vi "Get DUT Setup Parameters.vi"(8 "error in (no error)":errorcluster, 11 "QPA Measurement in":refnum<class "QPA Measurement.lvclass">) -> (0 "error out":errorcluster, 3 "QPA Measurement out":refnum<class "QPA Measurement.lvclass">)   [LabVIEW 2016, in "QPA Measurement.lvlib" / "QPA Measurement.lvclass"]
uses:
  QPA Measurement.lvclass
  C:/Projects/STS/Common/Sequence Automation/Plugins/Measurement Interface.lvlibp/Measurement Interface.lvclass
  QPA Measurement.lvclass/QPA Measurement.ctl
  Controls/Parameter.ctl
  Plugins/Measurement Interface.lvlibp/Private Methods/Active Sequence File/Read Active Sequence File.vi
  Plugins/TestStand API Tools (TSAT).lvlibp/Sequence File Actions/TSAT Sequence File Actions.lvlib
  Plugins/TestStand API Tools (TSAT).lvlibp/Sequence Actions/TSAT Sequence Actions.lvlib
  Plugins/TestStand API Tools (TSAT).lvlibp/TSAT Utilities/TSAT Utilities.lvlib
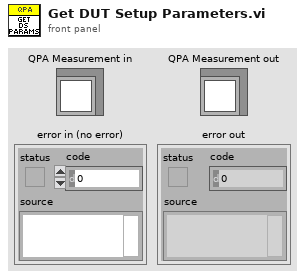
[diagram p1: front panel]
types:
  T1 = enum16{"Container", "String", "Boolean", "Number", "NamedType", "Reference", "Array", "Aperture Time"}
  T2 = typedef "QPA Measurement.lvlib/QPA Measurement.lvclass/Parameter.ctl" = cluster{"Name":string, "PropertyObject Type":enum16{"Container", "String", "Boolean", "Number", "NamedType", "Reference", "Array", "Aperture Time"}}
  T3 = enum16{"Container", "String", "Boolean", "Number", "NamedType", "Reference", "Array"}
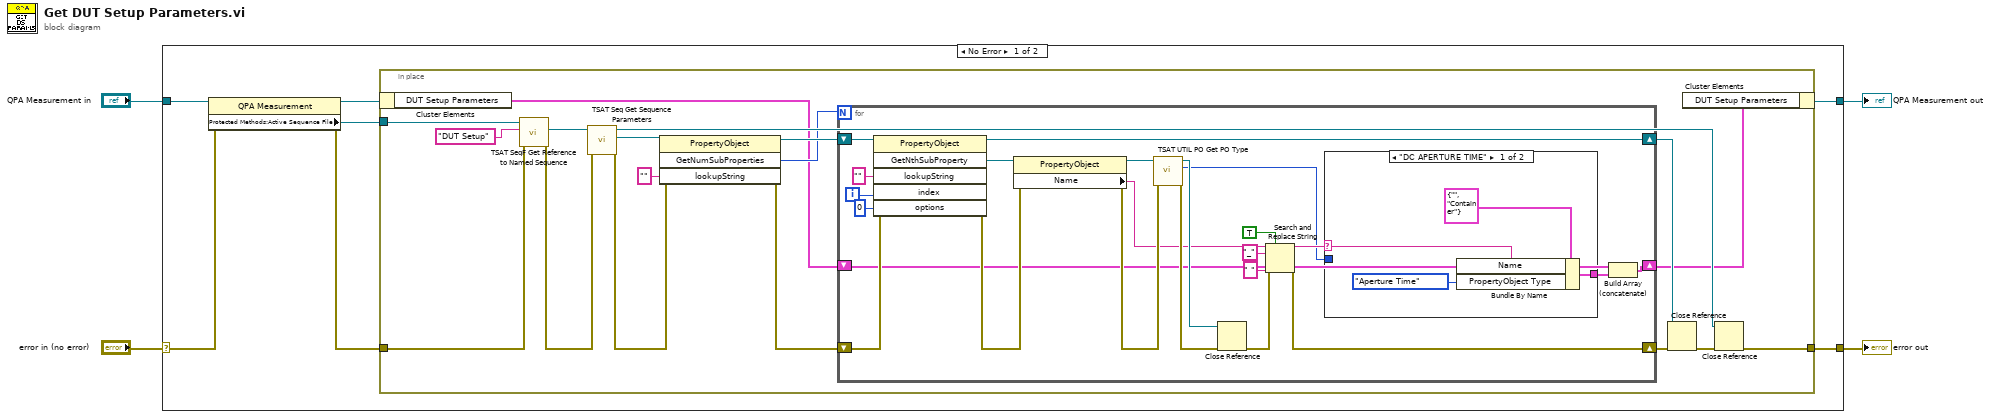
[diagram p0: block diagram]
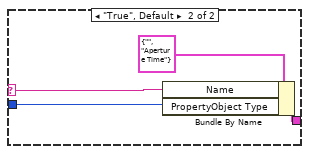
[diagram p2: hidden frame]
diagram:
  n1 = case shown="No Error" "error in (no error)" {
    selector: "error in (no error)" -> [w11 w62]
    tunnel: [w5 w62] -> w3
    tunnel: [w10 w61] -> w1
    tunnel: "QPA Measurement in" -> [w8 w61]
    frame No Error {
      n2 = property class="QPA Measurement"(reference=w8, error in=w11) -> (reference out=w7:refnum<class "QPA Measurement.lvclass">, error out=w9:errorcluster, "Protected Methods:Active Sequence File"=w6:refnum<k7>)
      n3 = in-place {
        in-place-border: w9 -> [w28]
        in-place-border: w6 -> [w29]
        in-place-border: [w16] -> w5
        n4 = in-place-cluster #1(w7) -> ("DUT Setup Parameters"=w13:T2[])
        n5 = call "TSAT SeqF Get Reference to Named Sequence.vi"("Error In"=w28, "Seqeunce to Retrieve"="DUT Setup", "Sequence File In"=w29) -> ("Error Out"=w25:errorcluster, "Named Sequence"=w26:refnum<k7>)  [unwired: 6 in, 1 out]
        n6 = call "TSAT Seq Get Sequence Parameters.vi"("Error in"=w25, "Sequence Reference In"=w26) -> ("Error out"=w23:errorcluster, "Parameters"=w24:refnum<k7>, "Sequence Reference Out"=w15:refnum<k7>)  [unwired: 7 in]
        n7 = invoke class="PropertyObject" method="GetNumSubProperties"(reference=w24, error in=w23, "lookupString"="") -> (reference out=w20:refnum<k7>, error out=w21:errorcluster, "GetNumSubProperties"=w14:i32)  [unwired: 1 in, 1 out]
        n8 = for {
          N: w14 -> [_]
          shift-right: [w37] -> w19
          shift-left: w21 -> [w52]
          shift-right: [w50] -> w17
          shift-left: w20 -> [w51]
          shift-right: [w31] -> w12
          shift-left: w13 -> [w30]
          i -> [w48]
          n9 = invoke class="PropertyObject" method="GetNthSubProperty"(reference=w51, error in=w52, "lookupString"="", "index"=w48, "options"=0) -> (reference out=w50:refnum<k7>, error out=w45:errorcluster, "GetNthSubProperty"=w46:refnum<k7>)  [unwired: 1 in, 3 out]
          n10 = property class="PropertyObject"(reference=w46, error in=w45) -> (reference out=w42:refnum<k7>, error out=w44:errorcluster, "Name"=w40:string)
          n11 = call "TSAT UTIL PO Get PO Type.vi"("error in (no error)"=w44, "PropertyObject In"=w42) -> ("error out"=w43:errorcluster, "PropertyObject Type"=w33:T3, "PropertyObject Out"=w41:refnum<k7>)  [unwired: 7 in]
          n12 = Close Reference(reference=w41, error in (no error)=w43) -> (error out=w38:errorcluster)
          n13 = Search and Replace String(replace all?=TRUE ("replace all? (F)"), input string=w40, search string="_", replace string=" " ("replace string (\"\")"), error in=w38) -> (result string=w34:string, error out=w37:errorcluster)  [unwired: 3 in, 2 out]
          n14 = case shown="\"DC APERTURE TIME\"" w34 {
            selector: w34 -> [w55 w58]
            tunnel: w33 -> [_ w57]
            tunnel: [w54 w59] -> w32
            frame "DC APERTURE TIME" {
              n15 = Bundle By Name(cluster=T2 {"Name"="", "PropertyObject Type"=enum."Container"} ("Parameter"), "Name"=w55, "PropertyObject Type"=T1."Aperture Time") -> (w54:T2)
            }
            frame "True", Default {
              n16 = Bundle By Name(cluster=T2 {"Name"="", "PropertyObject Type"=enum."Aperture Time"} ("Parameter"), "Name"=w58, "PropertyObject Type"=w57) -> (w59:T2)
            }
          }
          n17 = Build Array (concatenate)(w30, w32) -> (w31:T2[])
        }
        n18 = Close Reference(reference=w17, error in (no error)=w19) -> (error out=w18:errorcluster)
        n19 = in-place-cluster #1("DUT Setup Parameters"=w12) -> (w10:refnum<class "QPA Measurement.lvclass">)
        n20 = Close Reference(reference=w15, error in (no error)=w18) -> (error out=w16:errorcluster)
      }
    }
    frame Error {
    }
  }
  "error out" <- w3
  "QPA Measurement out" <- w1
